vi "FormatOpenHandshake.vi"(4 "Websocket Version":i32=13, 6 "Websocket Key":string="dGhlIHNhbXBsZSBub25jZQ==", 7 "Port (9090)":u16=9090) -> (2 "opening handshake":string)   [LabVIEW 2014, in "Websocket.lvlib"]
uses:
  Websocket.lvlib
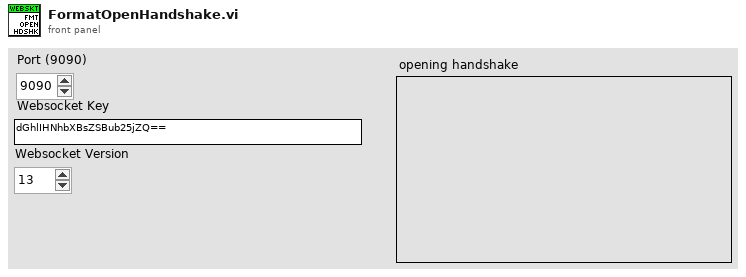
[diagram p1: front panel]
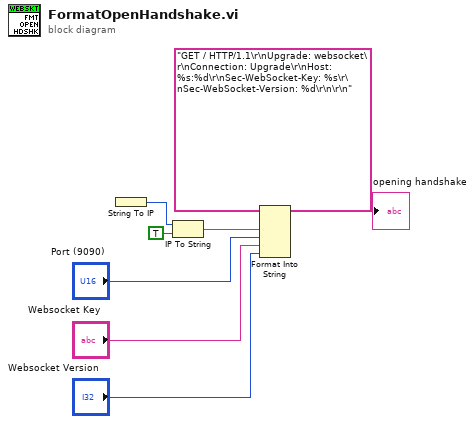
[diagram p0: block diagram]
diagram:
  n1 = String To IP() -> (0:w7:u32)  [unwired: 1 in]
  n2 = IP To String(1:TRUE ("dot notation? (F)"), 2:w7) -> (0:w5:string)
  n3 = Format Into String(format string="GET / HTTP/1.1\r\nUpgrade: websocket\r\nConnection: Upgrade\r\nHost: %s:%d\r\nSec-WebSocket-Key: %s\r\nSec-WebSocket-Version: %d\r\n\r\n" ("data in"), w5, "Port (9090)", "Websocket Key", "Websocket Version") -> (resulting string=→"opening handshake":string)  [unwired: 2 in, 1 out]
